vi "getJobOpeningsSeniorities.vi"(8 "errorIn":errorcluster, 11 "staisticsData":T1) -> (0 "errorOut":errorcluster, 3 "statistics":cluster{cluster{"X":dbl, "Y":dbl}[]}[](array[cluster]))   [LabVIEW 2025]
uses:
  control/statisticsData.ctl
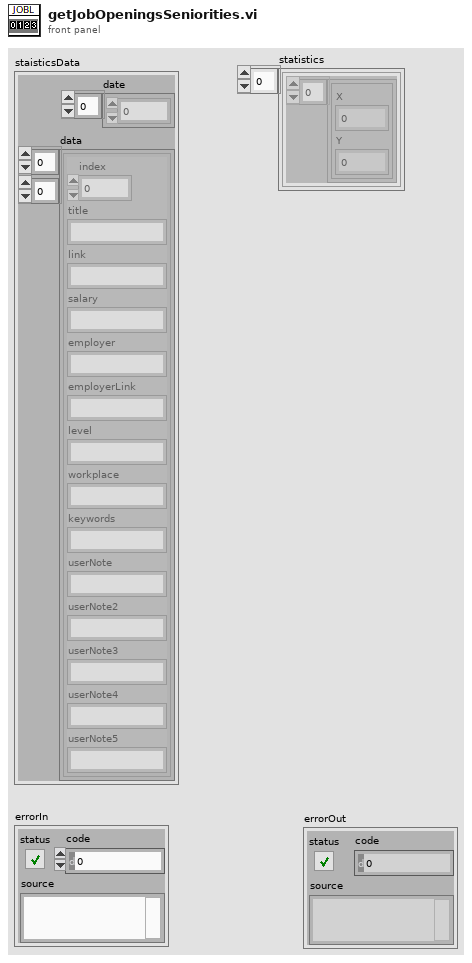
[diagram p1: front panel]
types:
  T1 = typedef "statisticsData.ctl" = cluster{"date":dbl[], "data":cluster{"index":i32, "title":string, "link":string, "salary":string, "employer":string, "employerLink":string, "level":string, "workplace":string, "keywords":string, "userNote":string, "userNote2":string, "userNote3":string, "userNote4":string, "userNote5":string}[][]}
  T2 = cluster{"index":i32, "title":string, "link":string, "salary":string, "employer":string, "employerLink":string, "level":string, "workplace":string, "keywords":string, "userNote":string, "userNote2":string, "userNote3":string, "userNote4":string, "userNote5":string}[][]
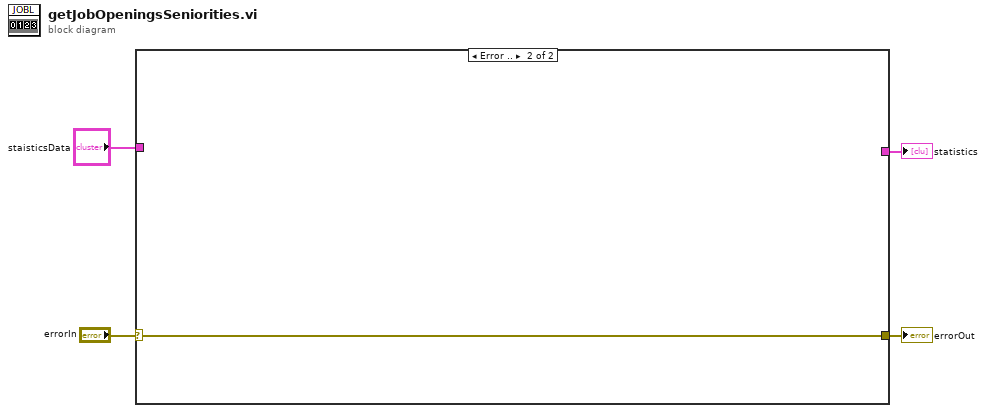
[diagram p0: block diagram]
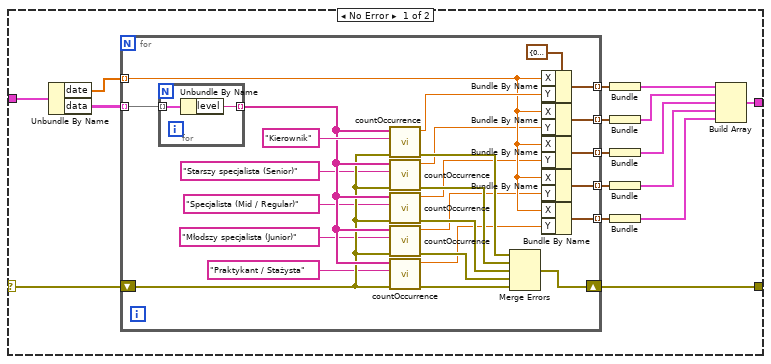
[diagram p2: hidden frame]
diagram:
  n1 = case shown="Error .." "errorIn" {
    selector: "errorIn" -> [w14 w49]
    tunnel: [w20 _] -> w4
    tunnel: "staisticsData" -> [w15 _]
    tunnel: [w5 w49] -> w1
    frame No Error {
      n2 = Unbundle By Name(w15) -> ("date"=w16:dbl[], "data"=w17:T2)
      n3 = for {
        tunnel: w16 -> [w33] mode=indexing
        tunnel: w17 -> [w46] mode=indexing
        tunnel: [w45] -> w18 mode=indexing
        shift-right: [w36] -> w5
        shift-left: w14 -> [w40]
        tunnel: [w28] -> w13 mode=indexing
        tunnel: [w27] -> w12 mode=indexing
        tunnel: [w26] -> w11 mode=indexing
        tunnel: [w25] -> w10 mode=indexing
        w34 = cluster{"X":dbl, "Y":dbl} {"X"=0.0, "Y"=0.0}
        n4 = for {
          tunnel: w46 -> [w48] mode=indexing
          tunnel: [w47] -> w42 mode=indexing
          n5 = Unbundle By Name(w48) -> ("level"=w47:string)
        }
        n6 = call "countOccurrence.vi"("errorIn"=w40, "keyword"="Kierownik", "dataArray"=w42) -> ("errorOut"=w35:errorcluster, "amount"=w44:dbl)  [unwired: 7 in]
        n7 = call "countOccurrence.vi"("errorIn"=w40, "keyword"="Starszy specjalista (Senior)", "dataArray"=w42) -> ("errorOut"=w37:errorcluster, "amount"=w29:dbl)  [unwired: 7 in]
        n8 = call "countOccurrence.vi"("errorIn"=w40, "keyword"="Specjalista (Mid / Regular)", "dataArray"=w42) -> ("errorOut"=w38:errorcluster, "amount"=w30:dbl)  [unwired: 7 in]
        n9 = call "countOccurrence.vi"("errorIn"=w40, "keyword"="Młodszy specjalista (Junior)", "dataArray"=w42) -> ("errorOut"=w39:errorcluster, "amount"=w31:dbl)  [unwired: 7 in]
        n10 = call "countOccurrence.vi"("errorIn"=w40, "keyword"="Praktykant / Stażysta", "dataArray"=w42) -> ("errorOut"=w41:errorcluster, "amount"=w32:dbl)  [unwired: 7 in]
        n11 = Merge Errors(w35, w37, w38, w39, w41) -> (w36:errorcluster)
        n12 = Bundle By Name(cluster=w34, "X"=w33, "Y"=w44) -> (w45:cluster{"X":dbl, "Y":dbl})
        n13 = Bundle By Name(cluster=w34, "X"=w33, "Y"=w29) -> (w28:cluster{"X":dbl, "Y":dbl})
        n14 = Bundle By Name(cluster=w34, "X"=w33, "Y"=w30) -> (w27:cluster{"X":dbl, "Y":dbl})
        n15 = Bundle By Name(cluster=w34, "X"=w33, "Y"=w31) -> (w26:cluster{"X":dbl, "Y":dbl})
        n16 = Bundle By Name(cluster=w34, "X"=w33, "Y"=w32) -> (w25:cluster{"X":dbl, "Y":dbl})
      }
      n17 = Bundle(w18) -> (w19:cluster{cluster{"X":dbl, "Y":dbl}[]})  [unwired: 1 in]
      n18 = Bundle(w13) -> (w9:cluster{cluster{"X":dbl, "Y":dbl}[]})  [unwired: 1 in]
      n19 = Bundle(w12) -> (w8:cluster{cluster{"X":dbl, "Y":dbl}[]})  [unwired: 1 in]
      n20 = Bundle(w11) -> (w7:cluster{cluster{"X":dbl, "Y":dbl}[]})  [unwired: 1 in]
      n21 = Bundle(w10) -> (w6:cluster{cluster{"X":dbl, "Y":dbl}[]})  [unwired: 1 in]
      n22 = Build Array(w19, w9, w8, w7, w6) -> (w20:cluster{cluster{"X":dbl, "Y":dbl}[]}[])
    }
    frame Error {
    }
  }
  "statistics" <- w4
  "errorOut" <- w1
